vi "Open-session.vi"(8 "error in (no error)":errorcluster, 9 "Camport":u32, 10 "Framegrabber board":i32, 11 "PF_MV1-D1312-240 in":refnum<class "PF_MV1-D1312-240.lvclass">) -> (0 "error out":errorcluster, 2 "IMAQ Session":refnum<k11>, 3 "PF_MV1-D1312-240 out":refnum<class "PF_MV1-D1312-240.lvclass">)   [LabVIEW 2013, in "CameraVision.lvlib" / "PF_MV1-D1312-240.lvclass"]
uses:
  PF_MV1-D1312-240.lvclass
  Camera.lvclass/Camera.ctl
  Write IMAQ Session.vi
  <userlib>/Photonfocus Toolkit/Photonfocus_Toolkit.lvlib
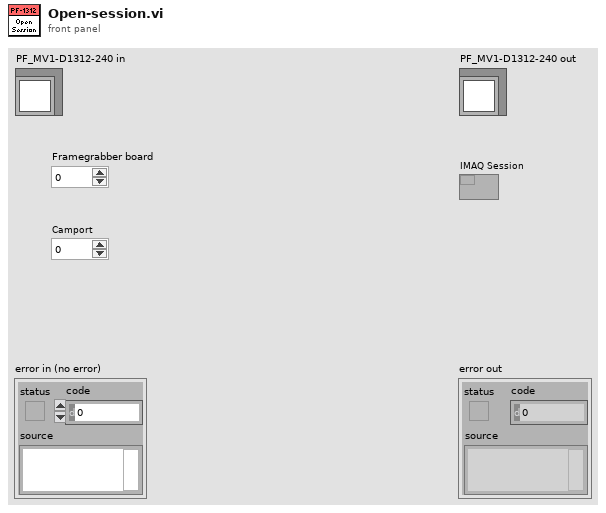
[diagram p1: front panel]
types:
  T1 = cluster{"Max. offset X":i32, "Max. offset Y":i32, "Offset step size X":i32, "Offset step size Y":i32}
  T2 = cluster{"Max. width":i32, "Max. height":i32, "Step size width":dbl, "Min. width":i32, "Min. height":i32, "Step size height":dbl}
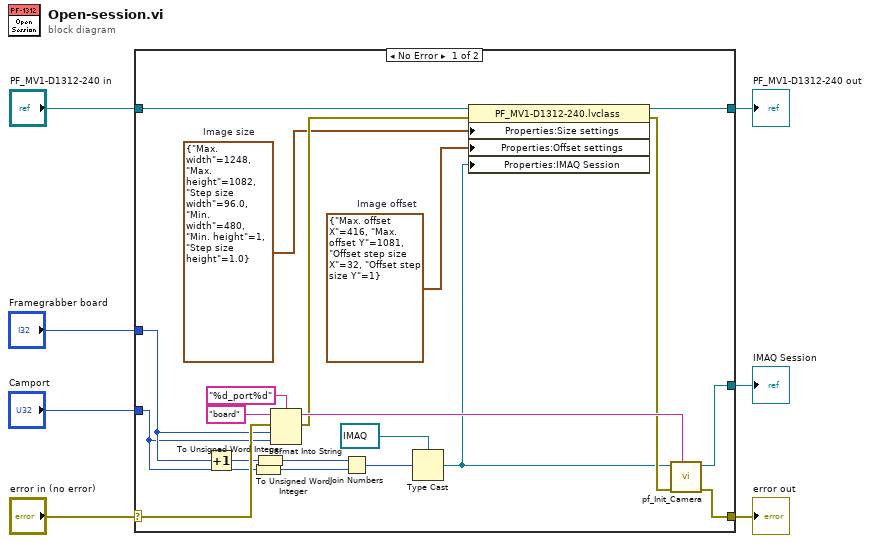
[diagram p0: block diagram]
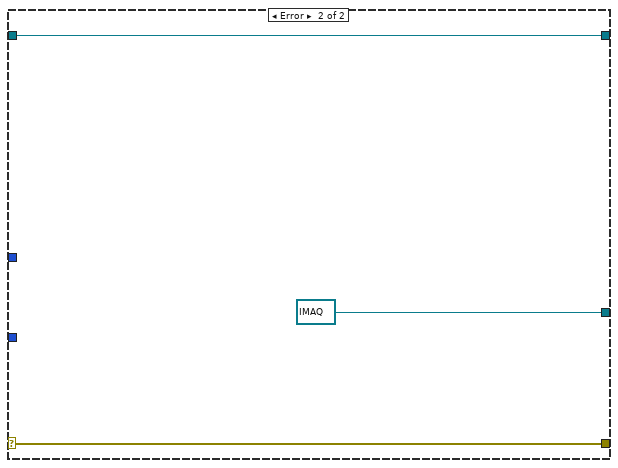
[diagram p2: hidden frame]
diagram:
  n1 = case shown="No Error" "error in (no error)" {
    selector: "error in (no error)" -> [w24 w30]
    tunnel: [w23 w30] -> w6
    tunnel: [w16 w29] -> w4
    tunnel: "PF_MV1-D1312-240 in" -> [w27 w29]
    tunnel: "Framegrabber board" -> [w19 _]
    tunnel: "Camport" -> [w18 _]
    tunnel: [w25 refnum<k11> refnum ("IMAQ Session out")] -> w1
    frame No Error {
      w11 = T1 {"Max. offset X"=416, "Max. offset Y"=1081, "Offset step size X"=32, "Offset step size Y"=1}  # Image offset
      w12 = T2 {"Max. width"=1248, "Max. height"=1082, "Step size width"=96.0, "Min. width"=480, "Min. height"=1, "Step size height"=1.0}  # Image size
      n2 = Increment(x=w19) -> (x+1=w10:i32)
      n3 = To Unsigned Word Integer(number=w18) -> (unsigned 16bit integer=w8:u16)
      n4 = To Unsigned Word Integer(number=w10) -> (unsigned 16bit integer=w9:u16)
      n5 = Format Into String(format string="%d_port%d", initial string="board", error in=w24, w19, w18) -> (resulting string=w21:string, error out=w15:errorcluster)
      n6 = Join Numbers(hi=w9, lo=w8) -> ((hi.lo)=w20:u32)
      n7 = Type Cast(type=refnum<k11> refnum ("IMAQ Session in"), x=w20) -> (*(type *) &x=w13:refnum<k11>)
      n8 = property class="PF_MV1-D1312-240.lvclass"(reference=w27, error in=w15, "Properties:Size settings"=w12, "Properties:Offset settings"=w11, "Properties:IMAQ Session"=w13) -> (reference out=w16:refnum<class "PF_MV1-D1312-240.lvclass">, error out=w14:errorcluster)
      n9 = call <userlib>:"pf_Init_Camera.vi"("Interface Name"=w21, "error in (no error)"=w14, "IMAQ Session in"=w13) -> ("error out"=w23:errorcluster, "IMAQ Session out"=w25:refnum<k11>)  [unwired: 1 in, 6 out]
    }
    frame Error {
    }
  }
  "error out" <- w6
  "PF_MV1-D1312-240 out" <- w4
  "IMAQ Session" <- w1
